vi "Error cyc Times.vi"(8 "error in (no error)":errorcluster, 11 "Status in":bool) -> (0 "error out":errorcluster, 1 "Numeric":i32, 2 "Cys Status":bool, 3 "Status out":bool)   [LabVIEW 2014]
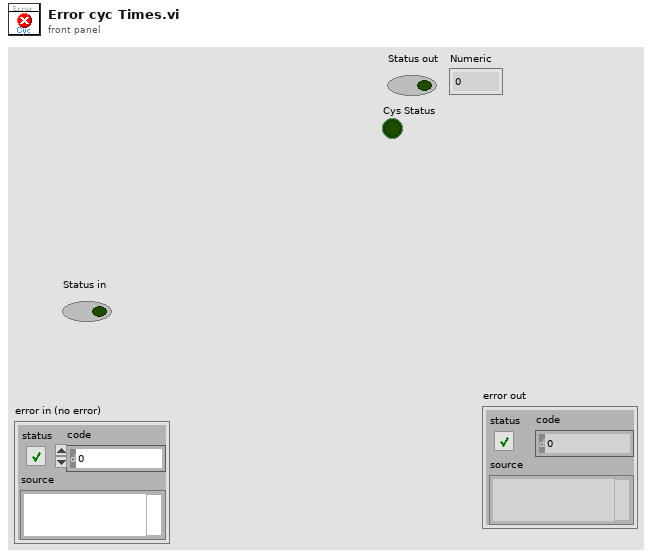
[diagram p1: front panel]
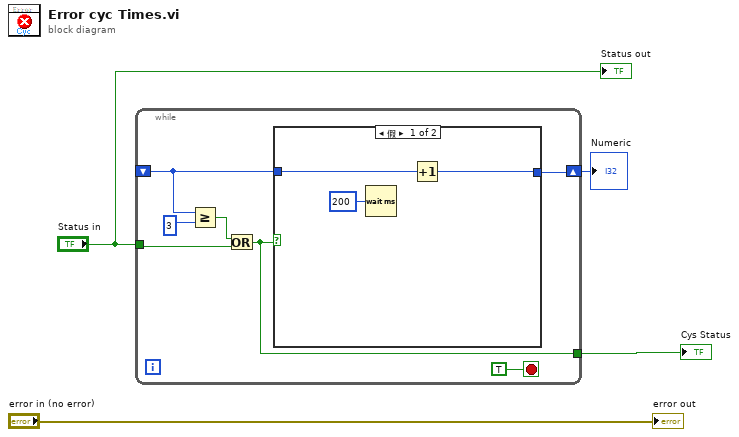
[diagram p0: block diagram]
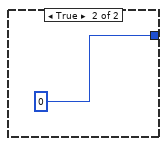
[diagram p2: hidden frame]
diagram:
  n1 = while {
    tunnel: "Status in" -> [w10]
    shift-right: [w9] -> w1
    shift-left: _ -> [w6]
    tunnel: [w5] -> w2
    stop <- TRUE stop-if-true
    n2 = Greater Or Equal?(x=w6, y=3) -> (x >= y?=w7:bool)
    n3 = Or(x=w7, y=w10) -> (x .or. y?=w5:bool)
    n4 = case shown="假" w5 {
      tunnel: [w13 0] -> w9
      tunnel: w6 -> [w14 _]
      frame False {
        n5 = Wait (ms)(milliseconds to wait=u32 200) -> ()  [unwired: 1 out]
        n6 = Increment(x=w14) -> (x+1=w13:i32)
      }
      frame True {
      }
    }
  }
  "Cys Status" <- w2
  "Numeric" <- w1
  "error out" <- "error in (no error)"
  "Status out" <- "Status in"
